vi "find_term_objects_pos_and_refs.vi"(0 "VI Ref In":refnum<vi>, 11 "error in (no error)":errorcluster) -> (3 "Last Function":refnum<vi>, 4 "VI Ref Out":refnum<vi>, 6 "Last Control Position":cluster{"Left":i32, "Top":i32}, 8 "Last StrCnst Refnum":refnum<vi>, 10 "Last Function Position":cluster{"Left":i32, "Top":i32}, 15 "error out":errorcluster)   [LabVIEW 2018]
uses:
  <vilib>/Utility/miscctls.llb/LVPositionTypeDef.ctl
  <vilib>/Utility/traverseref.llb/TRef TravTarget.ctl
  <vilib>/Utility/traverseref.llb/VI Scripting - Traverse.lvlib
panel:
  out "Last String Constant Position":T1
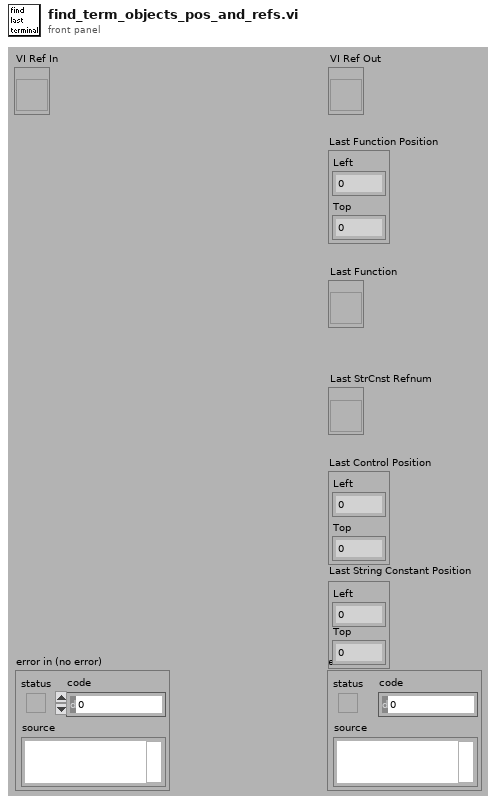
[diagram p1: front panel]
types:
  T1 = typedef "LVPositionTypeDef.ctl" = cluster{"Left":i32, "Top":i32}
  T2 = typedef "TRef TravTarget.ctl" = enum16{"FP", "BD", "Other"}
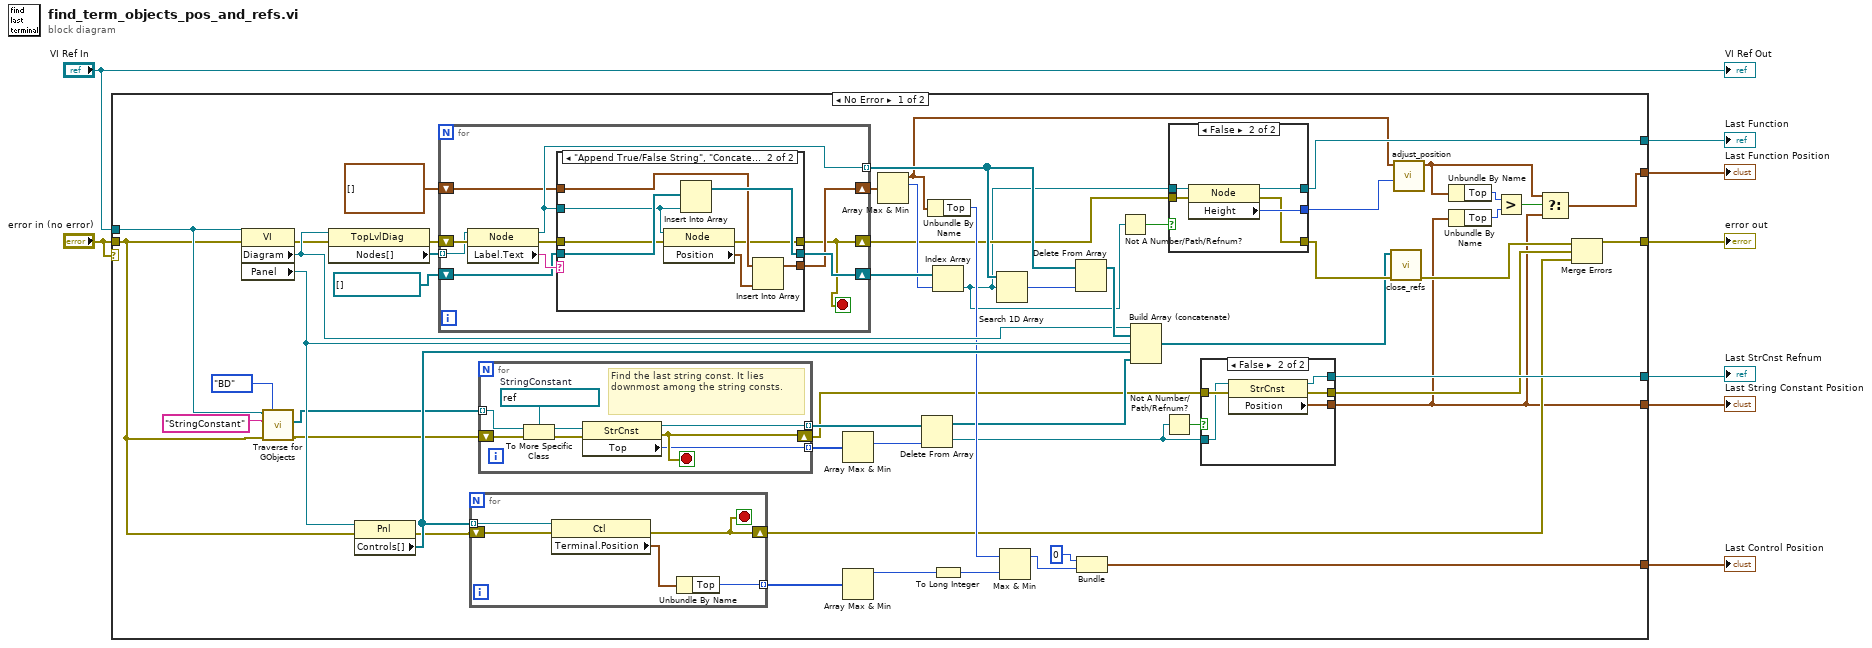
[diagram p0: block diagram]
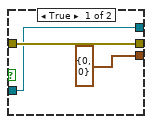
[diagram p2: hidden frame]
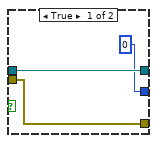
[diagram p3: hidden frame]
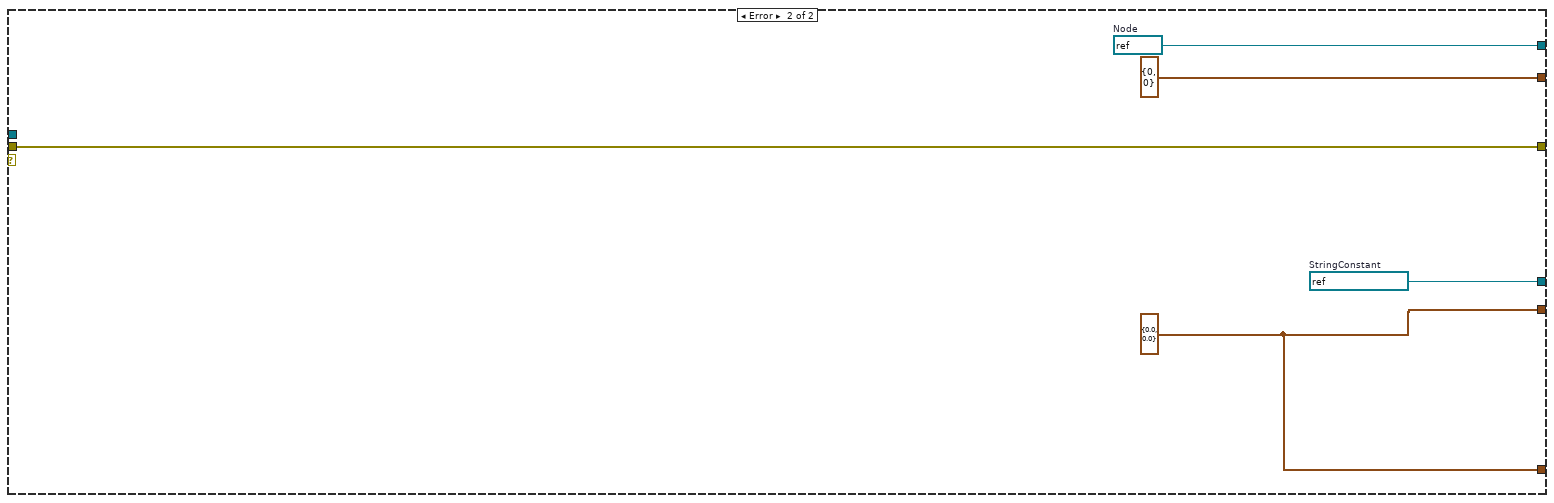
[diagram p5: hidden frame]
diagram:
  n1 = case shown="No Error" "error in (no error)" {
    tunnel: "error in (no error)" -> [w11 w117]
    tunnel: [w29 w117] -> w8
    tunnel: "VI Ref In" -> [w13 _]
    tunnel: [w21 cluster{"Left":i32, "Top":i32} {"Left"=0, "Top"=0}] -> w6
    tunnel: [w48 w113] -> w5
    tunnel: [w47 w115] -> w3
    tunnel: [w34 w114] -> w2
    tunnel: [w22 w113] -> w1
    frame No Error {
      n2 = property class="VI"(reference=w13, error in=w11) -> (error out=w54:errorcluster, "Diagram"=w55:refnum<vi>, "Panel"=w52:refnum<vi>)  [unwired: 1 out]
      n3 = call <vilib>:"Traverse for GObjects.vi"("Traverse Target"=TRef_TravTarget."BD", "error in (no error)"=w11, "Class Name"="StringConstant", "VI Refnum"=w13) -> ("error out"=w10:errorcluster, "References"=w9:refnum<vi>[])  [unwired: 4 in, 2 out]
      n4 = property class="TopLvlDiag"(reference=w55, error in=w54) -> (error out=w53:errorcluster, "Nodes[]"=w16:refnum<vi>[])  [unwired: 1 out]
      n5 = property class="Pnl"(reference=w52, error in=w11) -> (error out=w32:errorcluster, "Controls[]"=w51:refnum<vi>[])  [unwired: 1 out]
      n6 = for {
        tunnel: w16 -> [w88] mode=indexing
        shift-right: [w94] -> w60
        shift-left: refnum<vi>[] [] -> [w95]
        tunnel: [w93] -> w58 mode=indexing
        shift-right: [w91] -> w61
        shift-left: cluster{"Left":i32, "Top":i32}[] [] ("Array 4") -> [w92]
        shift-right: [w87] -> w46
        shift-left: w53 -> [w90]
        stop <- w87 stop-if-true
        n7 = property class="Node"(reference=w88, error in=w90) -> (reference out=w93:refnum<vi>, error out=w89:errorcluster, "Label.Text"=w96:string)
        n8 = case shown="\"Append True/False String\", \"Concatenate Strings\", \"Format Into String\", \"Pick Line\"" w96 {
          tunnel: w93 -> [_ w105]
          tunnel: w95 -> [w99 w107]
          tunnel: [w99 w106] -> w94
          tunnel: w92 -> [w98 w103]
          tunnel: [w98 w102] -> w91
          tunnel: w89 -> [w97 w101]
          tunnel: [w97 w100] -> w87
          frame Default {
          }
          frame "Append True/False String", "Concatenate Strings", "Format Into String", "Pick Line" {
            n9 = property class="Node"(reference=w105, error in=w101) -> (error out=w100:errorcluster, "Position"=w104:T1)  [unwired: 1 out]
            n10 = Insert Into Array(array=w107, new element=w105) -> (w106:refnum<vi>[])  [unwired: 1 in]
            n11 = Insert Into Array(array=w103, new element=w104) -> (w102:cluster{"Left":i32, "Top":i32}[])  [unwired: 1 in]
          }
        }
      }
      n12 = for {
        tunnel: w51 -> [w112] mode=indexing
        shift-right: [w108] -> w28
        shift-left: w32 -> [w111]
        tunnel: [w109] -> w20 mode=indexing
        stop <- w108 stop-if-true
        n13 = property class="Ctl"(reference=w112, error in=w111) -> (error out=w108:errorcluster, "Terminal.Position"=w110:T1)  [unwired: 1 out]
        n14 = Unbundle By Name(w110) -> ("Top"=w109:i32)
      }
      n15 = for {
        tunnel: w9 -> [w77] mode=indexing
        shift-right: [w72] -> w33
        shift-left: w10 -> [w76]
        tunnel: [w71] -> w38 mode=indexing
        tunnel: [w73] -> w37 mode=indexing
        stop <- w72 stop-if-true
        w78 = refnum<vi> refnum  # StringConstant
        # "Find the last string const. It lies downmost among the string consts."
        n16 = To More Specific Class(target class=w78, reference=w77, error in=w76) -> (specific class reference=w75:refnum<vi>, error out=w74:errorcluster)
        n17 = property class="StrCnst"(reference=w75, error in=w74) -> (reference out=w73:refnum<vi>, error out=w72:errorcluster, "Top"=w71:i32)
      }
      n18 = Array Max & Min(array=w38) -> (max index (indices)=w36:i32)  [unwired: 3 out]
      n19 = Array Max & Min(array=w20) -> (max value=w19:i32)  [unwired: 3 out]
      n20 = Array Max & Min(array=w61) -> (max value=w41:cluster{"Left":i32, "Top":i32}, max index (indices)=w59:i32)  [unwired: 2 out]
      n21 = Delete From Array(array=w37, index=w36) -> (deleted portion=w15:refnum<vi>, array with subset deleted=w35:refnum<vi>[])  [unwired: 1 in]
      n22 = Unbundle By Name(w41) -> ("Top"=w50:i32)
      n23 = Index Array(array=w60, index=w59) -> (element=w45:refnum<vi>)
      n24 = To Long Integer(number=w19) -> (32bit integer=w49:i32)
      n25 = Search 1D Array(1D array=w58, element=w45) -> (index of element=w57:i32)  [unwired: 1 out]
      n26 = Max & Min(x=w50, y=w49) -> (max(x,y)=w17:i32)  [unwired: 1 out]
      n27 = Delete From Array(array=w58, index=w57) -> (array with subset deleted=w56:refnum<vi>[])  [unwired: 1 in, 1 out]
      n28 = Bundle("Left"=0, w17) -> (w48:cluster{"Left":i32, i32})  [unwired: 1 out]
      n29 = Not A Number/Path/Refnum?(number/path/refnum=w45) -> (NaN/Path/Refnum?=w44:bool)
      n30 = Build Array (concatenate)(w55, w56, w52, w51, w35) -> (w42:refnum<vi>[])
      n31 = Not A Number/Path/Refnum?(number/path/refnum=w15) -> (NaN/Path/Refnum?=w27:bool)
      n32 = case shown="False" w44 {
        tunnel: w45 -> [w81 w86]
        tunnel: [w81 w85] -> w47
        tunnel: [u32 0 ("Height") w84] -> w40
        tunnel: w46 -> [w79 w83]
        tunnel: [w79 w82] -> w43
        frame True {
        }
        frame False {
          n33 = property class="Node"(reference=w86, error in=w83) -> (reference out=w85:refnum<vi>, error out=w82:errorcluster, "Height"=w84:u32)
        }
      }
      n34 = case shown="False" w27 {
        tunnel: [w64 w70] -> w34
        tunnel: w33 -> [w65 w69]
        tunnel: [w65 w68] -> w30
        tunnel: [T1 {"Left"=0, "Top"=0} ("Position") w67] -> w22
        tunnel: w15 -> [w64 w66]
        frame True {
        }
        frame False {
          n35 = property class="StrCnst"(reference=w66, error in=w69) -> (reference out=w70:refnum<vi>, error out=w68:errorcluster, "Position"=w67:T1)
        }
      }
      n36 = call "close_refs.vi"("error in"=w43, "Refs[]  In"=w42) -> ("error out"=w31:errorcluster)  [unwired: 9 out]
      n37 = call "adjust_position.vi"("Y Offset"=w40, "Position In"=w41) -> ("Position Out"=w23:cluster{"Left":i32, "Top":i32})  [unwired: 1 in, 8 out]
      n38 = Unbundle By Name(w23) -> ("Top"=w26:i32)
      n39 = Unbundle By Name(w22) -> ("Top"=w25:i32)
      n40 = Greater?(x=w26, y=w25) -> (0:w24:bool)
      n41 = Select(t=w23, s=w24, f=w22) -> (s? t:f=w21:T1)
      n42 = Merge Errors(w31, w30, w28) -> (w29:errorcluster)
    }
    frame Error {
      w114 = refnum<vi> refnum  # StringConstant
      w115 = refnum<vi> refnum  # Node
      w113 = cluster{"Left":dbl, "Top":dbl} {"Left"=0.0, "Top"=0.0}
    }
  }
  "Last Function Position" <- w6
  "Last Control Position" <- w5
  "error out" <- w8
  "Last Function" <- w3
  "Last StrCnst Refnum" <- w2
  "Last String Constant Position" <- w1
  "VI Ref Out" <- "VI Ref In"
